vi "Convert to Previous version of LabVIEW.vi"(6 "Error Handling":T1(ring), 7 "Previous Version":string(combo)="9.0", 8 "error in (no error)":errorcluster, 10 "Destination for down converted files.":path, 11 "Folder of LabVIEW files":path) -> (0 "error out":errorcluster, 3 "Path out":path)   [LabVIEW 2023]
doc: "This VI will convert a folder of VIs to a previous (selectable) version of LabVIEW."
uses:
  <userlib>/_OpenG.lib/file/file.llb/Strip Path Extension - Path__ogtk.vi
  <userlib>/_OpenG.lib/file/file.llb/openg_file.lvlib
panel:
  out "Convert Fails":path[](array[path])
  out "ALL Errors":errorcluster[](array[cluster])
  out "Path":path
  out "Progress":string
  # "Overview:This VI will convert a folder of VIs to a previous (selectable) version of LabVIEW.\nRequirements: LabVIEW 2012 or compatible\nInstructions:\n1.choose the Previous Version\n2.Run VI"
  # "Mass Compile for previous version"
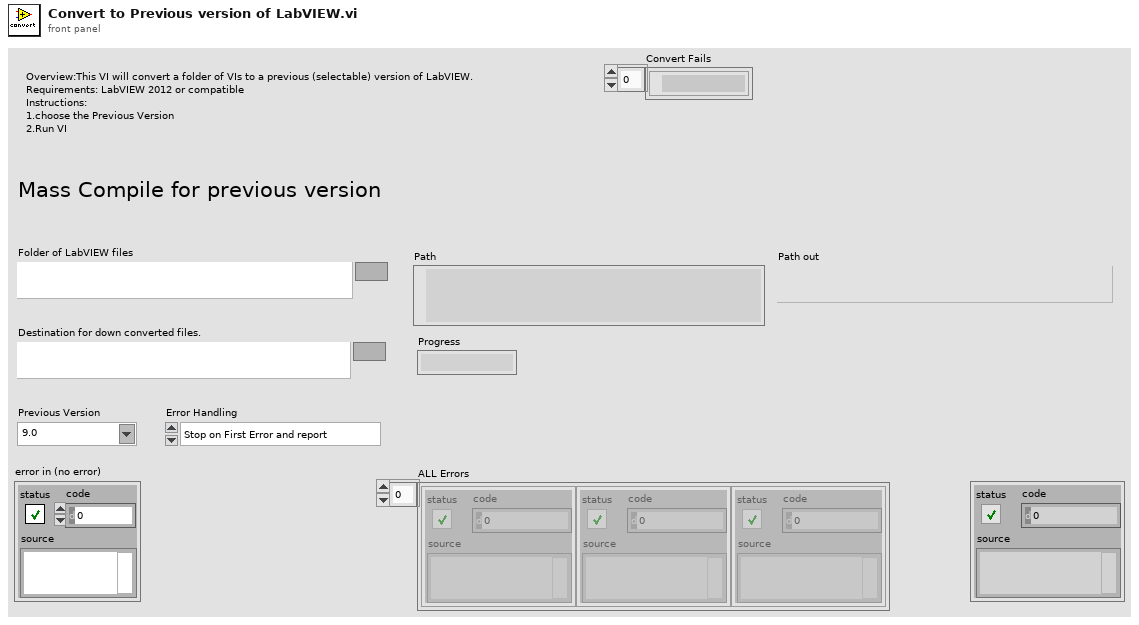
[diagram p1: front panel]
types:
  T1 = enum16{"Stop on First Error and report", "Continue on Error and Report", "Clear all Errors"}
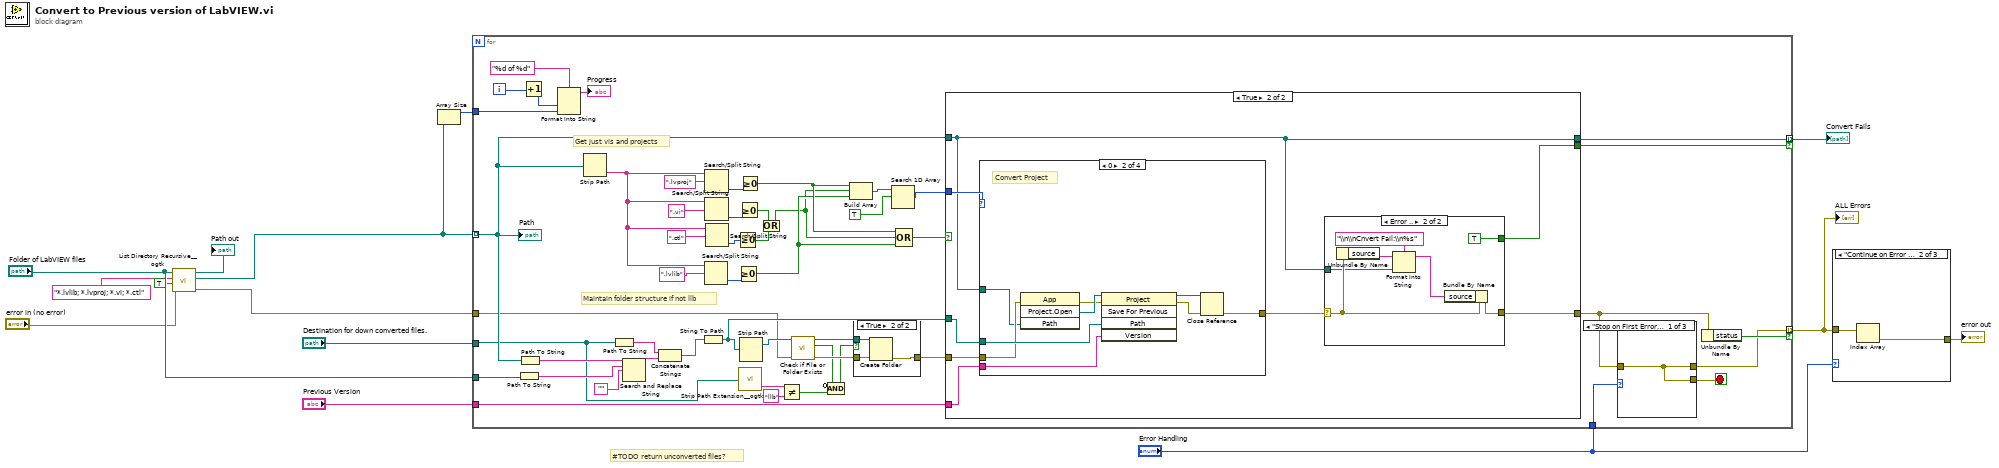
[diagram p0: block diagram]
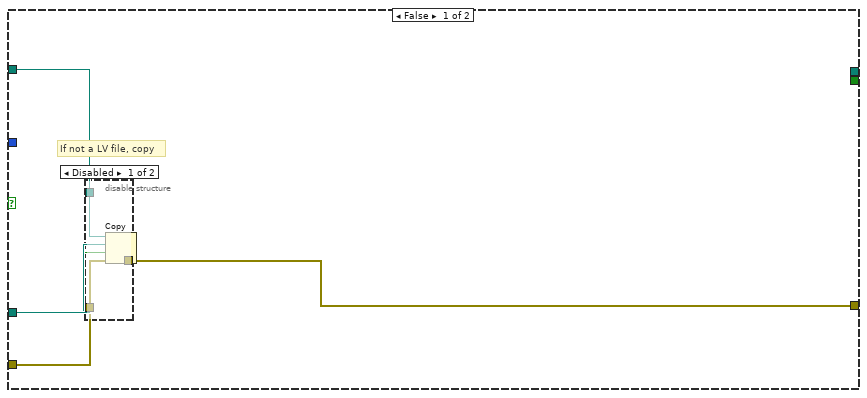
[diagram p2: hidden frame]
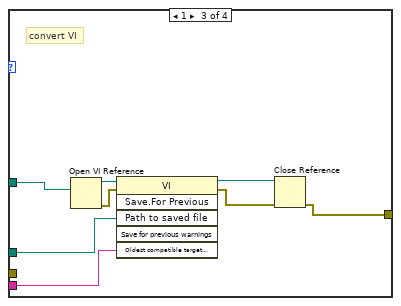
[diagram p5: hidden frame]
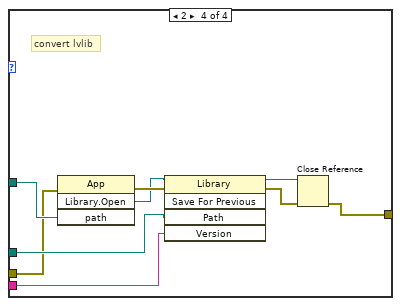
[diagram p6: hidden frame]
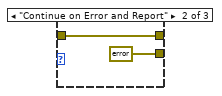
[diagram p9: hidden frame]
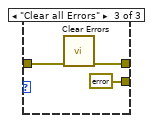
[diagram p10: hidden frame]
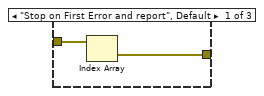
[diagram p11: hidden frame]
diagram:
  # "#TODO return unconverted files?"
  n1 = call <userlib>:"List Directory Recursive__ogtk.vi"("error in (no error)"="error in (no error)", "Treat llb files as directories? (FALSE)"=TRUE, "pattern"="*.lvlib; *.lvproj; *.vi; *.ctl", "Path"="Folder of LabVIEW files") -> ("error out"=w5:errorcluster, "file paths"=w10:path[], "dup Path"=→"Path out":path)  [unwired: 4 in, 1 out]
  n2 = Array Size(array=w10) -> (size(s)=w12:i32)
  n3 = for {
    tunnel: w10 -> [w52] mode=indexing
    tunnel: "Destination for down converted files." -> [w34]
    tunnel: "Folder of LabVIEW files" -> [w65]
    tunnel: "Previous Version" -> [w57]
    tunnel: w12 -> [w49]
    tunnel: [w20] -> w4 mode=indexing if=w21
    tunnel: "Error Handling" -> [w22]
    tunnel: w5 -> [w18]
    tunnel: [w16] -> w1 mode=indexing if=w15
    i -> [w51]
    stop <- w17 stop-if-true
    # "Get just vis and projects"
    # "Maintain folder structure if not llb"
    n4 = Path To String(path=w65) -> (string=w63:string)
    n5 = Path To String(path=w52) -> (string=w64:string)
    n6 = Increment(x=w51) -> (x+1=w50:i32)
    n7 = Format Into String(format string="%d of %d" ("search string"), w50, w49) -> (resulting string=→"Progress":string)  [unwired: 2 in, 1 out]
    n8 = Strip Path(path=w52) -> (name=w28:string)  [unwired: 1 out]
    n9 = Path To String(path=w34) -> (string=w61:string)
    n10 = Search and Replace String(input string=w64, search string=w63, replace string="") -> (result string=w60:string)  [unwired: 5 in, 3 out]
    n11 = Concatenate Strings(w61, w60) -> (w59:string)
    n12 = String To Path(string=w59) -> (path=w58:path)
    n13 = Search/Split String(string=w28, search string/char (-)=".lvlib" ("search string")) -> (offset of match=w37:i32)  [unwired: 1 in, 2 out]
    n14 = Search/Split String(string=w28, search string/char (-)=".lvproj" ("search string")) -> (offset of match=w39:i32)  [unwired: 1 in, 2 out]
    n15 = Search/Split String(string=w28, search string/char (-)=".vi" ("search string")) -> (offset of match=w35:i32)  [unwired: 1 in, 2 out]
    n16 = Search/Split String(string=w28, search string/char (-)=".ctl" ("search string")) -> (offset of match=w26:i32)  [unwired: 1 in, 2 out]
    n17 = Greater Or Equal To 0?(x=w26) -> (x >= 0?=w25:bool)
    n18 = Greater Or Equal To 0?(x=w37) -> (x >= 0?=w44:bool)
    n19 = Greater Or Equal To 0?(x=w35) -> (x >= 0?=w24:bool)
    n20 = Greater Or Equal To 0?(x=w39) -> (x >= 0?=w45:bool)
    n21 = call-poly <userlib>:"Strip Path Extension__ogtk.vi"("path"=w34) -> ("extension"=w33:string)  [unwired: 1 out]
    n22 = Strip Path(path=w58) -> (stripped path=w55:path)  [unwired: 1 out]
    n23 = Or(x=w24, y=w25) -> (x .or. y?=w23:bool)
    n24 = Not Equal?(x=w33, y="llb") -> (x != y?=w31:bool)
    n25 = call <vilib>:"Check if File or Folder Exists.vi"("error in (no error)"=w18, "path"=w55) -> ("error out"=w54:errorcluster, "file or folder exists?"=w30:bool, "dup path"=w46:path)  [unwired: 7 in]
    n26 = Compound Arithmetic op=AND(invert w30, w31) -> (w29:bool)
    n27 = Build Array(w45, w23, w44) -> (w43:bool[])
    n28 = case shown="True" w29 {
      tunnel: [w118 w121] -> w56
      tunnel: w54 -> [w118 w120]
      tunnel: w46 -> [_ w119]
      frame False {
      }
      frame True {
        n29 = Create Folder(path (use dialog)=w119, error in=w120) -> (error out=w121:errorcluster)  [unwired: 1 in, 2 out]
      }
    }
    n30 = Search 1D Array(1D array=w43, element=TRUE ("x >= 0?")) -> (index of element=w41:i32)  [unwired: 1 in]
    n31 = Compound Arithmetic op=OR(w45, w23, w44) -> (w53:bool)
    n32 = case shown="True" w53 {
      tunnel: [w66 w77] -> w19
      tunnel: w58 -> [w68 w80]
      tunnel: w57 -> [_ w82]
      tunnel: w56 -> [w67 w81]
      tunnel: w52 -> [w69 w76]
      tunnel: w41 -> [_ w79]
      tunnel: [_ w76] -> w16
      tunnel: [_ w75] -> w15
      frame False {
        # "If not a LV file, copy"
        n33 = disable-structure shown="Disabled" {
          disable-tunnel: w69 -> [w74 _]
          disable-tunnel: w68 -> [w73 _]
          disable-tunnel: w67 -> [w72 _]
          disable-tunnel: [w70 _] -> w66
          frame Disabled {
            n34 = Copy(8:w72, 9:TRUE ("overwrite (F)"), 10:w73, 11:w74) -> (0:w70:errorcluster)  [unwired: 1 in, 2 out]
          }
          frame Enabled {
          }
        }
      }
      frame True {
        n35 = case shown="0" w79 {
          tunnel: w80 -> [_ w89 w99 w105]
          tunnel: w76 -> [_ w85 w97 w107]
          tunnel: [w83 w84 w94 w103] -> w78
          tunnel: w82 -> [_ w87 w93 w104]
          tunnel: w81 -> [w83 w86 _ w102]
          frame -1, Default {
          }
          frame 0 {
            # "Convert Project"
            n36 = invoke class="App" method="Project.Open"(error in=w86, "Path"=w85) -> (error out=w90:errorcluster, "Project:Open"=w92:refnum<vi>)  [unwired: 2 in, 2 out]
            n37 = invoke class="Project" method="Save For Previous"(reference=w92, error in=w90, "Path"=w89, "Version"=w87) -> (reference out=w91:refnum<vi>, error out=w88:errorcluster)  [unwired: 1 in, 3 out]
            n38 = Close Reference(reference=w91, error in (no error)=w88) -> (error out=w84:errorcluster)
          }
          frame 1 {
            # "convert VI"
            n39 = Open VI Reference(vi path=w97) -> (vi reference=w98:refnum<vi>, error out=w100:errorcluster)  [unwired: 5 in]
            n40 = invoke class="VI" method="Save.For Previous"(reference=w98, error in=w100, "Path to saved file"=w99, "Oldest compatible target version"=w93) -> (reference out=w96:refnum<vi>, error out=w95:errorcluster)  [unwired: 2 in, 4 out]
            n41 = Close Reference(reference=w96, error in (no error)=w95) -> (error out=w94:errorcluster)
          }
          frame 2 {
            # "convert lvlib"
            n42 = invoke class="App" method="Library.Open"(error in=w102, "path"=w107) -> (error out=w109:errorcluster, "Open Library"=w106:refnum<vi>)  [unwired: 2 in, 2 out]
            n43 = invoke class="Library" method="Save For Previous"(reference=w106, error in=w109, "Path"=w105, "Version"=w104) -> (reference out=w101:refnum<vi>, error out=w108:errorcluster)  [unwired: 1 in, 3 out]
            n44 = Close Reference(reference=w101, error in (no error)=w108) -> (error out=w103:errorcluster)
          }
        }
        n45 = case shown="Error .." w78 {
          selector: w78 -> [w110 w117]
          tunnel: [w110 w116] -> w77
          tunnel: w76 -> [_ w114]
          tunnel: [_ TRUE] -> w75
          frame No Error {
          }
          frame Error {
            n46 = Unbundle By Name(w117) -> ("source"=w115:string)
            n47 = Format Into String(format string="\\n\\nCnvert Fail:\\n%s", initial string=w115, w114) -> (resulting string=w112:string)  [unwired: 1 in, 1 out]
            n48 = Bundle By Name(cluster=w117, "source"=w112) -> (w116:errorcluster)
          }
        }
      }
    }
    n49 = case shown="\"Stop on First Error and report\", Default" w22 {
      tunnel: [w122 w124 w126] -> w20
      tunnel: w19 -> [w122 w124 w127]
      tunnel: [w122 errorcluster {"status"=FALSE, "code"=0, "source"=""} ("error out") errorcluster {"status"=FALSE, "code"=0, "source"=""} ("error out")] -> w17
      frame "Stop on First Error and report", Default {
      }
      frame "Continue on Error and Report" {
      }
      frame "Clear all Errors" {
        n50 = call <vilib>:"Clear Errors.vi"("error in (no error)"=w127) -> ("error out"=w126:errorcluster)  [unwired: 5 in, 1 out]
      }
    }
    n51 = Unbundle By Name(w19) -> ("status"=w21:bool)
    "Path" <- w52
  }
  "ALL Errors" <- w4
  "Convert Fails" <- w1
  n52 = case shown="\"Continue on Error and Report\"" "Error Handling" {
    tunnel: w4 -> [w129 w130 _]
    tunnel: [w128 w131 _] -> w3
    frame "Stop on First Error and report", Default {
      n53 = Index Array(array=w129) -> (element=w128:errorcluster)  [unwired: 1 in]
    }
    frame "Continue on Error and Report" {
      n54 = Index Array(array=w130) -> (element=w131:errorcluster)  [unwired: 1 in]
    }
    frame "Clear all Errors" {
    }
  }
  "error out" <- w3
